vi "MeasurementItems_GetSingleChannel.vi"(8 "error in (no error)":errorcluster, 10 "#Channel (1..32768)":u16=1 min=1 max=32768, 11 "OXY_SCPI Reseource In":refnum<visa-resource-name>) -> (0 "error out":errorcluster, 1 "communication_data":T1, 2 "Channel Name":string, 3 "OXY_SCPI Reseource Out":refnum<visa-resource-name>)   [LabVIEW 2018, in "OXYGEN.lvlib"]
doc: "Query channel name of output item."
uses:
  OXYGEN.lvlib
  TypeDefs/Cluster_RawCommData.ctl
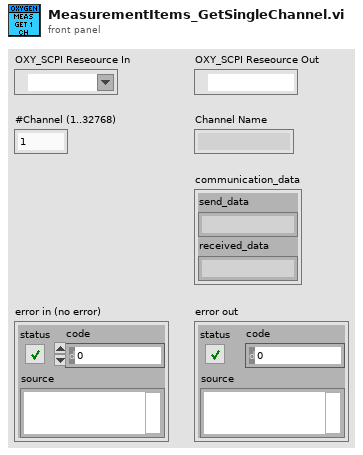
[diagram p1: front panel]
types:
  T1 = typedef "OXYGEN.lvlib/Cluster_RawCommData.ctl" = cluster{"send_data":string, "received_data":string}
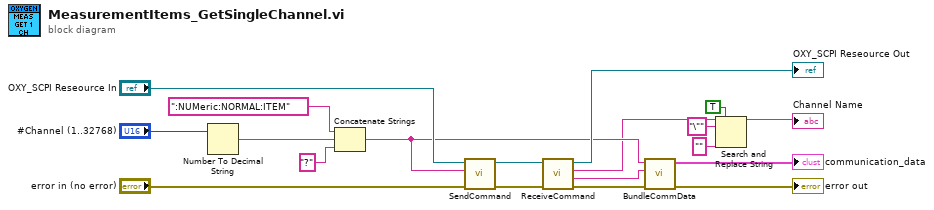
[diagram p0: block diagram]
diagram:
  n1 = Number To Decimal String(number="#Channel (1..32768)") -> (decimal integer string=w6:string)  [unwired: 1 in]
  n2 = Concatenate Strings(":NUMeric:NORMAL:ITEM" ("String to Send"), w6, "?" ("string")) -> (w8:string)
  n3 = call "SendCommand.vi"("error in (no error)"="error in (no error)", "String to Send"=w8, "OXY_SCPI Reseource In"="OXY_SCPI Reseource In") -> ("error out"=w19:errorcluster, "OXY_SCPI Reseource Out"=w18:refnum<visa-resource-name>)  [unwired: 7 in]
  n4 = call "ReceiveCommand.vi"("error in (no error)"=w19, "OXY_SCPI Reseource In"=w18) -> ("error out"=w14:errorcluster, "received Data with Header"=w12:string, "received Data"=w5:string, "OXY_SCPI Reseource Out"=→"OXY_SCPI Reseource Out":refnum<visa-resource-name>)  [unwired: 6 in]
  n5 = call "BundleCommData.vi"("error in (no error)"=w14, "received_data"=w12, "send_data"=w8) -> ("error out"=→"error out":errorcluster, "communication_data"=→"communication_data":T1)  [unwired: 7 in]
  n6 = Search and Replace String(replace all?=TRUE ("replace all? (F)"), input string=w5, search string="\"", replace string="" ("replace string (\"\")")) -> (result string=→"Channel Name":string)  [unwired: 4 in, 3 out]
